vi "Measurement UI.vi"() -> ()   [LabVIEW 2021, in "audio_acMeasurement.lvlib"]
uses:
  audio_acMeasurement.lvlib
panel:
  in  "MeasGraphs":T1(tab)
  out "FreqDomainGraph":cluster{"x0":dbl, "dx":dbl, "magnitude":dbl[]}(graph) caption="AC"
  out "TimeDomainGraph":waveform(dbl)(graph) caption="AC"
  in  "JSONFile":string
  out "Channel":string
  out "Spectrum":dbl[](array[numeric])
  out "df":dbl
  out "f0":dbl
  out "Time domain":dbl[](array[numeric])
  out "dt":dbl
  out "THD+N":dbl
  out "THD":dbl
  out "SNR":dbl
  out "Calculated amplitude":dbl
  out "Calculated frequency":dbl
  out "SFDR":dbl
  out "Dynamic range":dbl
  out "Gain error":dbl
  in  "Analog source resource name":string
  out "MeasTable":string[][](table)
  in  "Filename":string(combo)
  out "Sample rate":u32 caption="SAMPLE RATE" format="%#.6pHz"
  in  "Protocol capture channel":string="0L" caption="CHANNEL"
  in  "Protocol capture resource name":string caption="RESOURCE NAME"
  in  "Protocol settings":string="Protocol settings"
  in  "Analog source":string="Analog source "
  in  "Full scale range":dbl=3.16 caption="FULL SCALE RANGE" format="%.3pV"
  in  "Measurement settings":string="Measurement settings"
  in  "MeasSettingsOptions":i32(listbox)=-1
  in  "MeasSettings":bool
  in  "Protocol":u16(ring) caption="PROTOCOL" items=["I2S"]
  in  "DSGResourceName":tag caption="RESOURCE NAME"
  in  "Weighting filter":T2(ring) caption="WEIGHTING FILTER"
  in  "Number of words":u32=19200 caption="NUMBER OF WORDS"
  in  "Clock rate":u32=12288000 caption="CLOCK RATE" format="%#.6pHz"
  in  "Band stop":dbl=20000.0 caption="BAND STOP" format="%#_6pHz"
  in  "Band start":dbl=20.0 caption="BAND START" format="%#_6pHz"
  in  "Amplitude":dbl=-1.0 caption="AMPLITUDE" format="%#_6pdB"
  in  "Frequency":dbl=1000.0 caption="FREQUENCY" format="%#_6pHz"
  in  "Sensitivity":dbl=0.34762 caption="SENSITIVITY" format="%.5fFS/Pa"
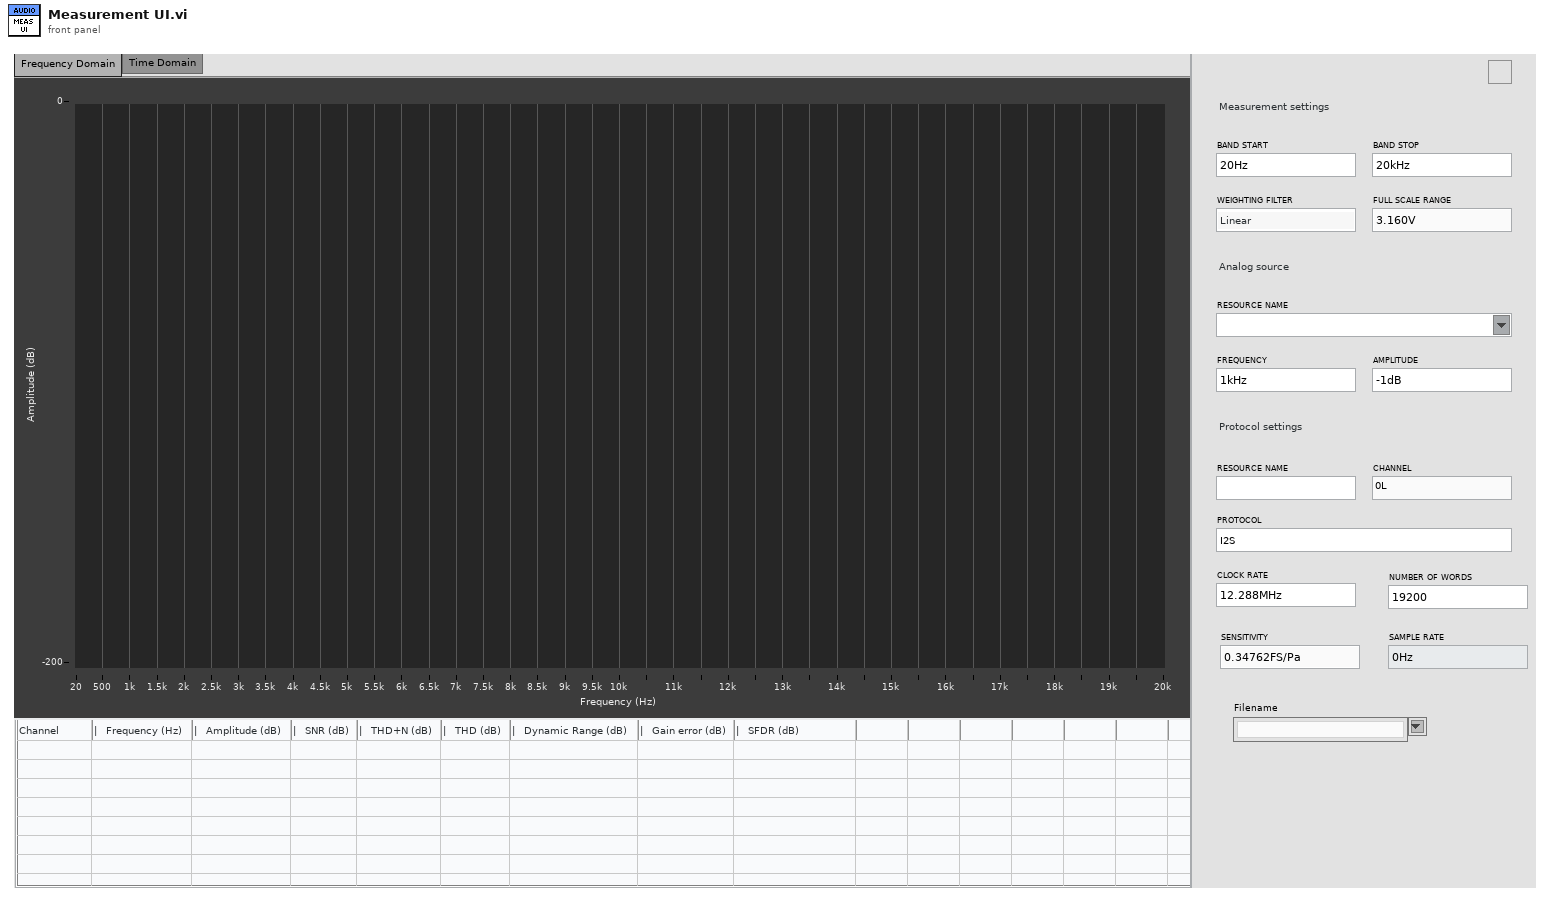
[diagram p1: front panel]
types:
  T1 = enum32{"Frequency Domain", "Time Domain", "Hidden Controls"}
  T2 = enum16{"Linear", "A-Weighting", "B-Weighting", "C-Weighting"}
  T3 = enum16{"open", "replace", "create", "open or create", "replace or create", "replace or create with confirmation"}
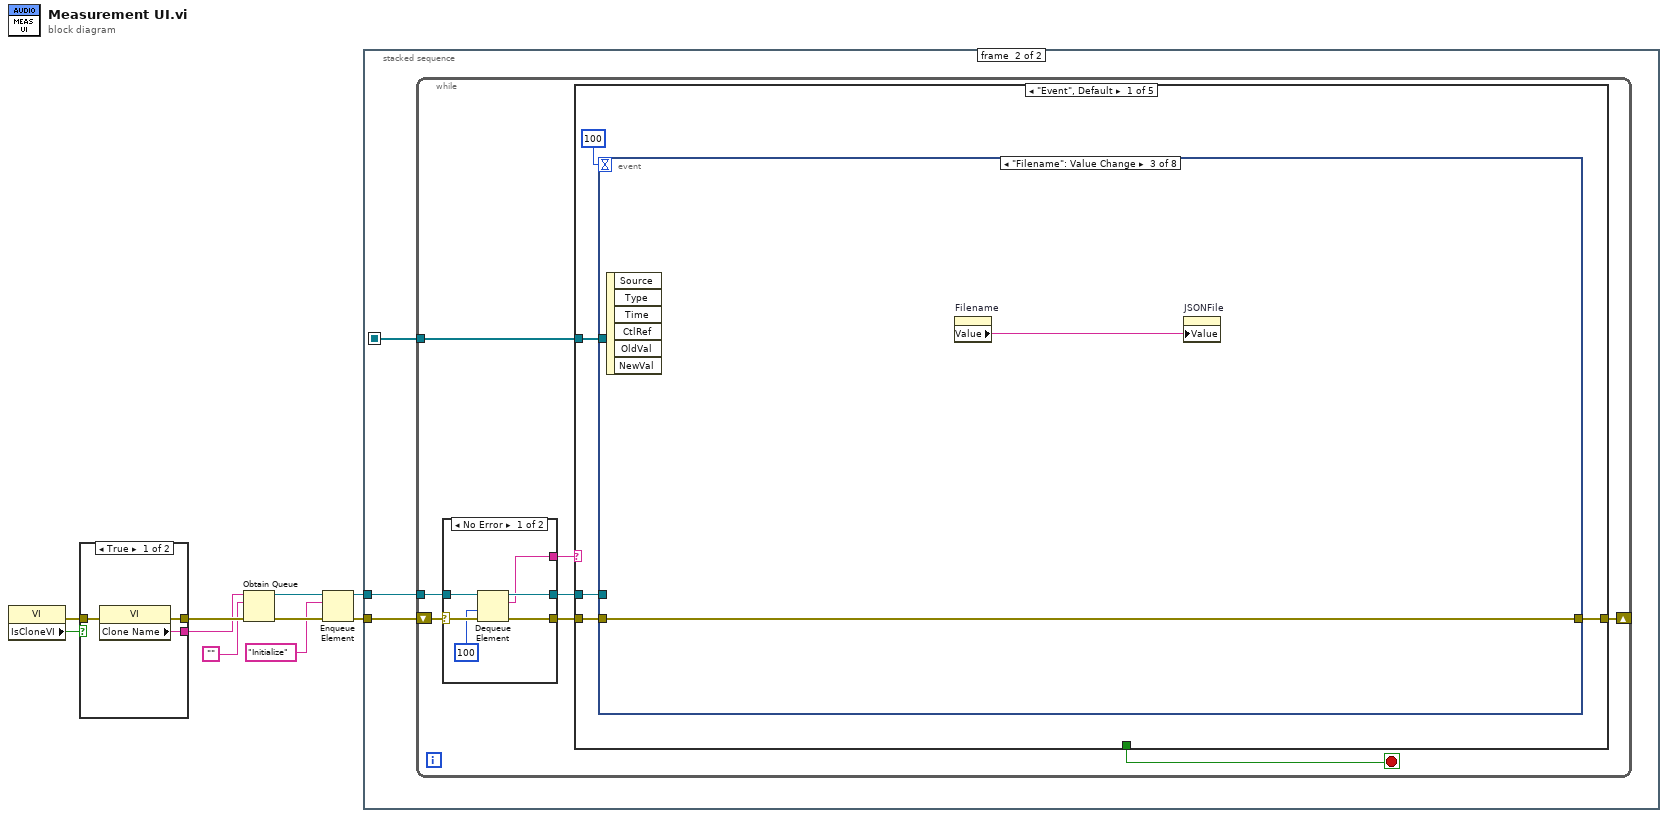
[diagram p0: block diagram]
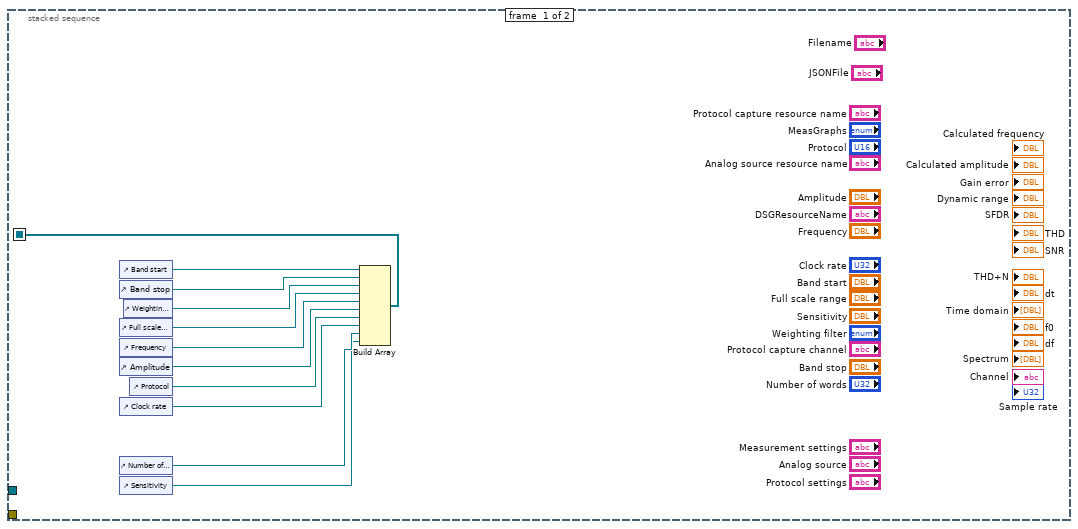
[diagram p2: hidden frame]
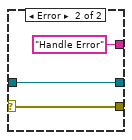
[diagram p3: hidden frame]
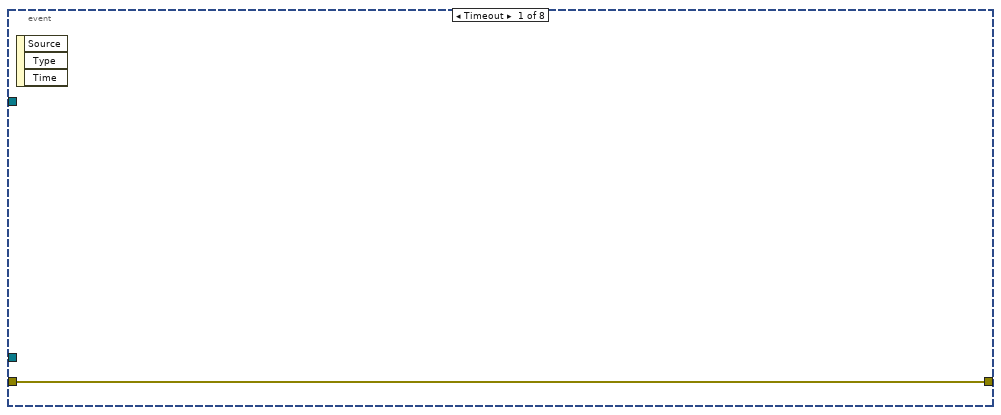
[diagram p4: hidden frame]
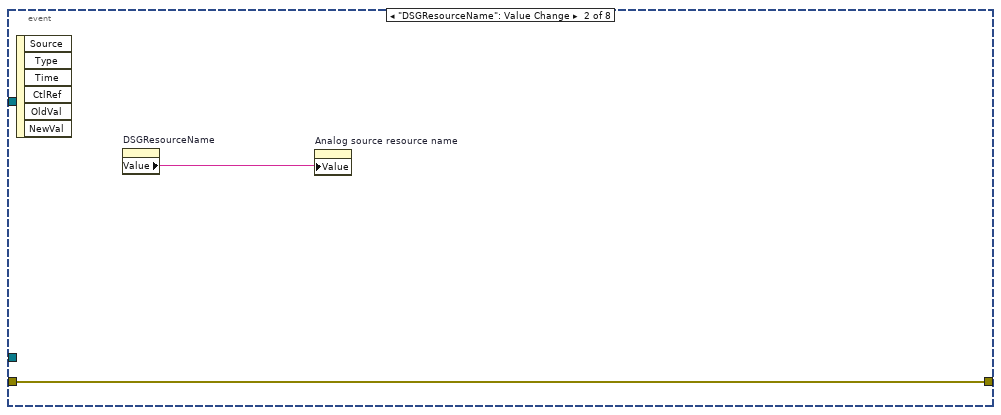
[diagram p5: hidden frame]
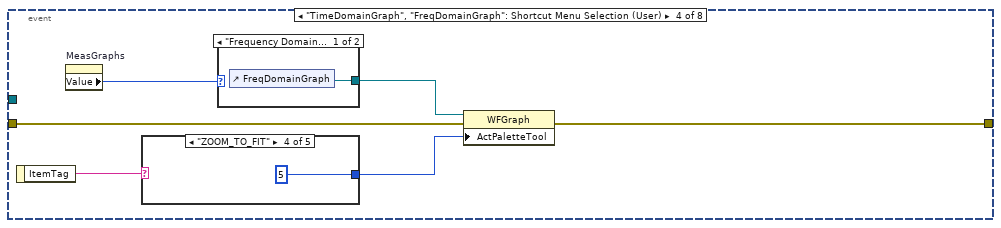
[diagram p6: hidden frame]
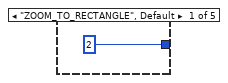
[diagram p7: hidden frame]
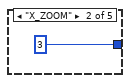
[diagram p8: hidden frame]
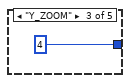
[diagram p9: hidden frame]
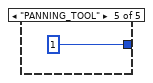
[diagram p10: hidden frame]
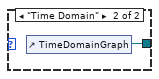
[diagram p11: hidden frame]
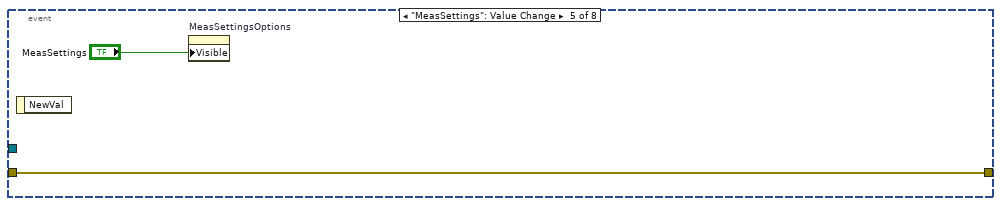
[diagram p12: hidden frame]
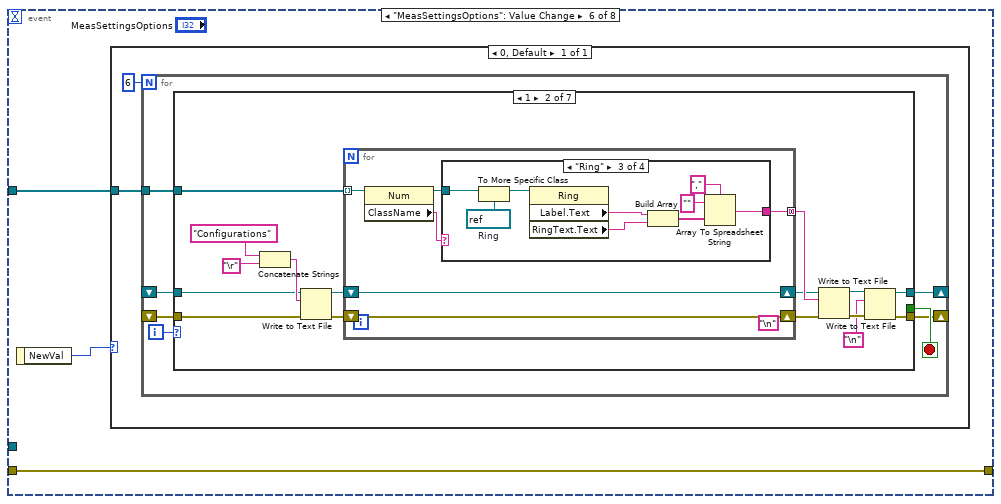
[diagram p13: hidden frame]
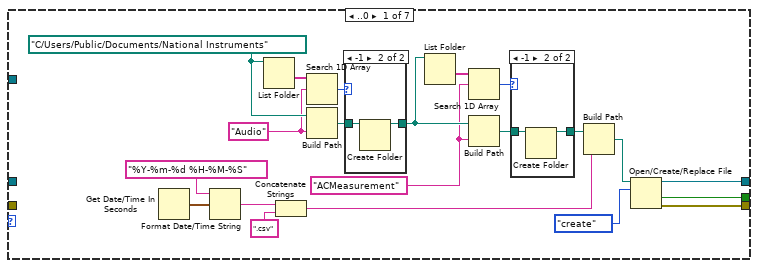
[diagram p14: hidden frame]
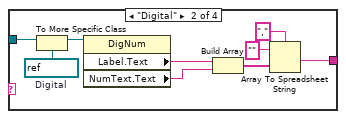
[diagram p18: hidden frame]
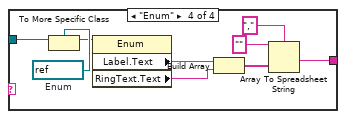
[diagram p19: hidden frame]
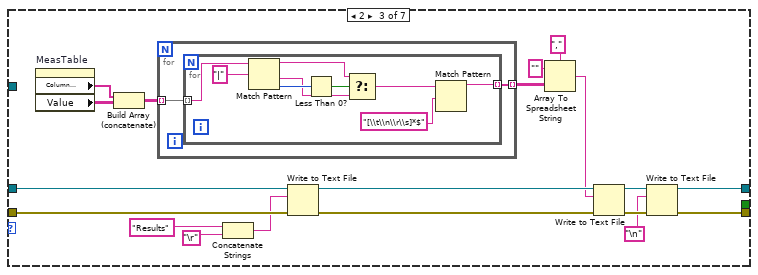
[diagram p20: hidden frame]
diagram:
  n1 = property class="VI"() -> (error out=w1:errorcluster, "IsCloneVI"=w2:bool)  [unwired: 2 in, 1 out]
  n2 = case shown="True" w2 {
    tunnel: [w13 w16] -> w10
    tunnel: [w12 w15] -> w9
    tunnel: w1 -> [w11 w14]
    frame True {
      n3 = property class="VI"(error in=w11) -> (error out=w13:errorcluster, "Clone Name"=w12:string)  [unwired: 1 in, 1 out]
    }
    frame False {
      n4 = property class="VI"(error in=w14) -> (error out=w16:errorcluster, "Name"=w15:string)  [unwired: 1 in, 1 out]
    }
  }
  n5 = Obtain Queue(name (unnamed)=w9, element data type="", error in (no error)=w10) -> (queue out=w6:refnum<queue>, error out=w8:errorcluster)  [unwired: 2 in, 1 out]
  n6 = Enqueue Element(queue=w6, element="Initialize", error in (no error)=w8) -> (queue out=w5:refnum<queue>, error out=w7:errorcluster)  [unwired: 1 in, 1 out]
  n7 = stacked-sequence {
    seq-local: [w24 _] -> [_ w28]
    tunnel: w7 -> [_ w30]
    tunnel: w5 -> [_ w29]
    frame #0 {
      n8 = control-ref of="Band start"() -> (w27:refnum<vi>)
      n9 = control-ref of="Band stop"() -> (w26:refnum<vi>)
      n10 = control-ref of="Full scale range"() -> (w23:refnum<vi>)
      n11 = control-ref of="Frequency"() -> (w20:refnum<vi>)
      n12 = control-ref of="Amplitude"() -> (w19:refnum<vi>)
      n13 = control-ref of="Clock rate"() -> (w22:refnum<vi>)
      n14 = control-ref of="Number of words"() -> (w18:refnum<vi>)
      n15 = control-ref of="Sensitivity"() -> (w17:refnum<vi>)
      n16 = control-ref of="Weighting filter"() -> (w25:refnum<vi>)
      n17 = control-ref of="Protocol"() -> (w21:refnum<vi>)
      n18 = Build Array(w27, w26, w25, w23, w20, w19, w21, w22, w18, w17) -> (w24:refnum<vi>[])
    }
    frame #1 {
      n19 = while {
        shift-right: [w33] -> _
        shift-left: w30 -> [w38]
        tunnel: w29 -> [w36]
        tunnel: w28 -> [w31]
        stop <- w32 stop-if-true
        n20 = case shown="No Error" w38 {
          selector: w38 -> [w44 w47]
          tunnel: [w43 w47] -> w37
          tunnel: w36 -> [w42 w46]
          tunnel: [w41 w46] -> w35
          tunnel: [w40 "Handle Error"] -> w34
          frame No Error {
            n21 = Dequeue Element(queue=w42, timeout in ms (-1)=100, error in (no error)=w44) -> (queue out=w41:refnum<queue>, element=w40:string, error out=w43:errorcluster)  [unwired: 1 out]
          }
          frame Error {
          }
        }
        n22 = case shown="\"Event\", Default" w34 {
          tunnel: w37 -> [w52 w283 w321 w336 w337]
          tunnel: w35 -> [w50 _ _ w334 _]
          tunnel: [w48 w283 w321 w331 w337] -> w33
          tunnel: [_ _ _ TRUE _] -> w32
          tunnel: w31 -> [w49 _ _ _ _]
          frame "Event", Default {
            n23 = event shown="[2] \"Filename\": Value Change" {
              selector: _ -> [_ _ _ _ _ _ _ _]
              dyn-events: _ -> [_ _ _ _ _ _ _ _]
              timeout: 100 -> [_ _ _ _ _ _ _ _]
              tunnel: w52 -> [w53 w54 w56 w59 w71 w75 w267 w273]
              tunnel: w50 -> [_ _ _ _ _ _ _ w271]
              tunnel: [_ _ _ _ w71 _ _ _] -> _
              tunnel: w49 -> [_ _ _ _ _ w73 _ _]
              tunnel: [w53 w54 w56 w60 _ w75 w267 w272] -> w48
              event Timeout {
                n24 = event-data() -> ()  [unwired: 1 in, 3 out]
              }
              event "DSGResourceName": Value Change {
                n25 = event-data() -> ()  [unwired: 1 in, 6 out]
                n26 = property on="DSGResourceName" class="DAQmxName"() -> ("Value"=w55:string)  [unwired: 2 in, 2 out]
                n27 = property on="Analog source resource name" class="Str"("Value"=w55) -> ()  [unwired: 2 in, 2 out]
              }
              event "Filename": Value Change {
                n28 = event-data() -> ()  [unwired: 1 in, 6 out]
                n29 = property on="Filename" class="CmbBox"() -> ("Value"=w57:string)  [unwired: 2 in, 2 out]
                n30 = property on="JSONFile" class="Str"("Value"=w57) -> ()  [unwired: 2 in, 2 out]
              }
              event "TimeDomainGraph", "FreqDomainGraph": Shortcut Menu Selection (User) {
                n31 = event-data() -> ("ItemTag"=w62:string)  [unwired: 1 in]
                n32 = property on="MeasGraphs" class="TabCtl (strict)"() -> ("Value"=w63:T1)  [unwired: 2 in, 2 out]
                n33 = case shown="\"ZOOM_TO_FIT\"" w62 {
                  tunnel: [2 3 4 5 1] -> w58
                  frame "ZOOM_TO_RECTANGLE", Default {
                  }
                  frame "X_ZOOM" {
                  }
                  frame "Y_ZOOM" {
                  }
                  frame "ZOOM_TO_FIT" {
                  }
                  frame "PANNING_TOOL" {
                  }
                }
                n34 = case shown="\"Frequency Domain\", Default" w63 {
                  tunnel: [w69 w70] -> w61
                  frame "Frequency Domain", Default {
                    n35 = control-ref of="FreqDomainGraph"() -> (w69:refnum<vi>)
                  }
                  frame "Time Domain" {
                    n36 = control-ref of="TimeDomainGraph"() -> (w70:refnum<vi>)
                  }
                }
                n37 = property class="WFGraph"(reference=w61, error in=w59, "ActPaletteTool"=w58) -> (error out=w60:errorcluster)  [unwired: 1 out]
              }
              event "MeasSettings": Value Change {
                n38 = event-data() -> ()  [unwired: 1 in, 1 out]
                n39 = property on="MeasSettingsOptions" class="LstBox (strict)"("Visible"="MeasSettings") -> ()  [unwired: 2 in, 2 out]
              }
              event "MeasSettingsOptions": Value Change {
                n40 = event-data() -> ("NewVal"=w74:i32)  [unwired: 1 in]
                n41 = case shown="0, Default" w74 {
                  tunnel: w73 -> [w76]
                  frame 0, Default {
                    n42 = for {
                      N: 6 -> [_]
                      shift-right: [w82] -> _
                      shift-left: _ -> [w81]
                      shift-right: [w80] -> _
                      shift-left: _ -> [w79]
                      tunnel: w76 -> [w78]
                      i -> [w84]
                      stop <- w83 stop-if-true
                      n43 = case shown="1" w84 {
                        tunnel: [w98 _ _ _ _ _ _] -> w83
                        tunnel: [w104 w124 w168 w195 w236 refnum<file> refnum ("refnum out") w266] -> w82
                        tunnel: w81 -> [_ w121 w179 w218 w237 w264 w266]
                        tunnel: [w97 w123 w167 w193 w235 w262 w265] -> w80
                        tunnel: w79 -> [_ w119 w178 w217 w238 w261 w265]
                        tunnel: w78 -> [_ w122 _ _ _ _ _]
                        frame ..0 {
                          w93 = "ACMeasurement" ("prompt")
                          w100 = "Audio" ("prompt")
                          w103 = path "C:/Users/Public/Documents/National Instruments" ("base path")
                          n44 = Get Date/Time In Seconds() -> (seconds since 1Jan1904=w90:timestamp)
                          n45 = Format Date/Time String(time format string (%c)="%Y-%m-%d %H-%M-%S", seconds (now)=w90) -> (date/time string=w89:string)  [unwired: 1 in]
                          n46 = List Folder(path=w103) -> (folder names=w101:string[])  [unwired: 3 in, 3 out]
                          n47 = Concatenate Strings(w89, ".csv" ("string")) -> (w86:string)
                          n48 = Search 1D Array(1D array=w101, element=w100) -> (index of element=w99:i32)  [unwired: 1 in]
                          n49 = Build Path(base path=w103, name or relative path=w100) -> (appended path=w102:path)
                          n50 = case shown="-1" w99 {
                            tunnel: w102 -> [w109 w111]
                            tunnel: [w109 w110] -> w94
                            frame Default {
                            }
                            frame -1 {
                              n51 = Create Folder(path (use dialog)=w111) -> (created path=w110:path)  [unwired: 2 in, 2 out]
                            }
                          }
                          n52 = List Folder(path=w94) -> (folder names=w96:string[])  [unwired: 3 in, 3 out]
                          n53 = Search 1D Array(1D array=w96, element=w93) -> (index of element=w95:i32)  [unwired: 1 in]
                          n54 = Build Path(base path=w94, name or relative path=w93) -> (appended path=w92:path)
                          n55 = case shown="-1" w95 {
                            tunnel: w92 -> [w106 w108]
                            tunnel: [w106 w107] -> w87
                            frame Default {
                            }
                            frame -1 {
                              n56 = Create Folder(path (use dialog)=w108) -> (created path=w107:path)  [unwired: 2 in, 2 out]
                            }
                          }
                          n57 = Build Path(base path=w87, name or relative path=w86) -> (appended path=w85:path)
                          n58 = Open/Create/Replace File(file path (use dialog)=w85, operation (0:open)=T3."create") -> (refnum out=w104:refnum<file>, cancelled=w98:bool, error out=w97:errorcluster)  [unwired: 4 in]
                        }
                        frame 1 {
                          (unwired) "\n"
                          n59 = Concatenate Strings("Configurations" ("format string"), "\r") -> (w125:string)
                          n60 = Write to Text File(file (use dialog)=w121, text=w125, error in=w119) -> (refnum out=w118:refnum<file>, error out=w120:errorcluster)  [unwired: 1 in, 1 out]
                          n61 = for {
                            tunnel: w122 -> [w129] mode=indexing
                            shift-right: [w133] -> w116
                            shift-left: w118 -> [w133]
                            shift-right: [w132] -> w115
                            shift-left: w120 -> [w132]
                            tunnel: [w131] -> w117 mode=concatenating
                            n62 = property class="Num"(reference=w129) -> (reference out=w130:refnum<vi>, "ClassName"=w128:string)  [unwired: 1 in, 1 out]
                            n63 = case shown="\"Ring\"" w128 {
                              tunnel: [_ w137 w147 w156] -> w131
                              tunnel: w130 -> [_ w135 w145 w160]
                              frame Default {
                              }
                              frame "Digital" {
                                w134 = refnum<vi> refnum  # Digital
                                n64 = To More Specific Class(target class=w134, reference=w135) -> (specific class reference=w136:refnum<vi>)  [unwired: 1 in, 1 out]
                                n65 = property class="DigNum"(reference=w136) -> ("Label.Text"=w142:string, "NumText.Text"=w141:string)  [unwired: 1 in, 2 out]
                                n66 = Build Array(w142, w141) -> (w138:string[])
                                n67 = Array To Spreadsheet String(delimiter (Tab)=",", array=w138, 3:"" ("format string")) -> (spreadsheet string=w137:string)
                              }
                              frame "Ring" {
                                w144 = refnum<vi> refnum  # Ring
                                n68 = To More Specific Class(target class=w144, reference=w145) -> (specific class reference=w146:refnum<vi>)  [unwired: 1 in, 1 out]
                                n69 = property class="Ring"(reference=w146) -> ("Label.Text"=w143:string, "RingText.Text"=w151:string)  [unwired: 1 in, 2 out]
                                n70 = Build Array(w143, w151) -> (w148:string[])
                                n71 = Array To Spreadsheet String(delimiter (Tab)=",", array=w148, 3:"" ("format string")) -> (spreadsheet string=w147:string)
                              }
                              frame "Enum" {
                                w159 = refnum<vi> refnum  # Enum
                                n72 = To More Specific Class(target class=w159, reference=w160) -> (specific class reference=w155:refnum<vi>)  [unwired: 1 in, 1 out]
                                n73 = property class="Enum"(reference=w155) -> ("Label.Text"=w154:string, "RingText.Text"=w153:string)  [unwired: 1 in, 2 out]
                                n74 = Build Array(w154, w153) -> (w152:string[])
                                n75 = Array To Spreadsheet String(delimiter (Tab)=",", array=w152, 3:"" ("format string")) -> (spreadsheet string=w156:string)
                              }
                            }
                          }
                          n76 = Write to Text File(file (use dialog)=w116, text=w117, error in=w115) -> (refnum out=w114:refnum<file>, error out=w113:errorcluster)  [unwired: 1 in, 1 out]
                          n77 = Write to Text File(file (use dialog)=w114, text="\n", error in=w113) -> (refnum out=w124:refnum<file>, error out=w123:errorcluster)  [unwired: 1 in, 1 out]
                        }
                        frame 2 {
                          n78 = property on="MeasTable" class="Tbl (strict)"() -> ("Column Headers[]"=w162:string[], "Value"=w161:string[][])  [unwired: 2 in, 2 out]
                          n79 = Build Array (concatenate)(w162, w161) -> (w176:string[][])
                          n80 = for {
                            tunnel: w176 -> [w181] mode=indexing
                            tunnel: [w180] -> w175 mode=indexing
                            n81 = for {
                              tunnel: w181 -> [w183] mode=indexing
                              tunnel: [w182] -> w180 mode=indexing
                              n82 = Match Pattern(string=w183, regular expression="|") -> (before substring=w187:string, after substring=w186:string, offset past match=w189:i32)  [unwired: 1 in, 1 out]
                              n83 = Less Than 0?(x=w189) -> (x < 0?=w188:bool)
                              n84 = Select(t=w187, s=w188, f=w186) -> (s? t:f=w185:string)
                              n85 = Match Pattern(string=w185, regular expression="[\\t\\n\\r\\s]*$") -> (before substring=w182:string)  [unwired: 1 in, 3 out]
                            }
                          }
                          n86 = Concatenate Strings("Results" ("element"), "\r") -> (w163:string)
                          n87 = Write to Text File(file (use dialog)=w179, text=w163, error in=w178) -> (refnum out=w177:refnum<file>, error out=w171:errorcluster)  [unwired: 1 in, 1 out]
                          n88 = Array To Spreadsheet String(delimiter (Tab)=",", array=w175, 3:"" ("format string")) -> (spreadsheet string=w172:string)
                          n89 = Write to Text File(file (use dialog)=w177, text=w172, error in=w171) -> (refnum out=w170:refnum<file>, error out=w169:errorcluster)  [unwired: 1 in, 1 out]
                          n90 = Write to Text File(file (use dialog)=w170, text="\n", error in=w169) -> (refnum out=w168:refnum<file>, error out=w167:errorcluster)  [unwired: 1 in, 1 out]
                        }
                        frame 3 {
                          n91 = property on="FreqDomainGraph" class="WFGraph (strict)"() -> ("Value"=w198:cluster{"x0":dbl, "dx":dbl, "magnitude":dbl[]})  [unwired: 2 in, 2 out]
                          n92 = Concatenate Strings("Frequency Domain" ("string"), "\r") -> (w215:string)
                          n93 = Build Array("Frequency (Hz)", "Amplitude (dB)") -> (w214:string[])
                          n94 = Write to Text File(file (use dialog)=w218, text=w215, error in=w217) -> (refnum out=w211:refnum<file>, error out=w210:errorcluster)  [unwired: 1 in, 1 out]
                          n95 = Unbundle By Name(w198) -> ("dx"=w202:dbl, "x0"=w203:dbl, "magnitude"=w201:dbl[])
                          n96 = Array To Spreadsheet String(delimiter (Tab)=",", array=w214, 3:"" ("format string")) -> (spreadsheet string=w209:string)
                          n97 = Write to Text File(file (use dialog)=w211, text=w209, error in=w210) -> (refnum out=w208:refnum<file>, error out=w207:errorcluster)  [unwired: 1 in, 1 out]
                          n98 = for {
                            tunnel: w201 -> [w222] mode=indexing
                            tunnel: w202 -> [w226]
                            tunnel: w203 -> [w224]
                            tunnel: [w219] -> w204 mode=indexing
                            i -> [w227]
                            n99 = Multiply(x=w227, y=w226) -> (x*y=w225:dbl)
                            n100 = Add(x=w225, y=w224) -> (x+y=w223:dbl)
                            n101 = Format Into String(w223) -> (resulting string=w220:string)  [unwired: 3 in, 1 out]
                            n102 = Format Into String(w222) -> (resulting string=w221:string)  [unwired: 3 in, 1 out]
                            n103 = Build Array(w220, w221) -> (w219:string[])
                          }
                          n104 = Array To Spreadsheet String(delimiter (Tab)=",", array=w204, 3:"" ("format string")) -> (spreadsheet string=w200:string)
                          n105 = Write to Text File(file (use dialog)=w208, text=w200, error in=w207) -> (refnum out=w197:refnum<file>, error out=w196:errorcluster)  [unwired: 1 in, 1 out]
                          n106 = Write to Text File(file (use dialog)=w197, text="\n", error in=w196) -> (refnum out=w195:refnum<file>, error out=w193:errorcluster)  [unwired: 1 in, 1 out]
                        }
                        frame 4 {
                          n107 = property on="TimeDomainGraph" class="WFGraph (strict)"() -> ("Value"=w234:waveform(dbl))  [unwired: 2 in, 2 out]
                          n108 = Concatenate Strings("Time Domain" ("string"), "\r") -> (w250:string)
                          n109 = Write to Text File(file (use dialog)=w237, text=w250, error in=w238) -> (refnum out=w247:refnum<file>, error out=w246:errorcluster)  [unwired: 1 in, 1 out]
                          n110 = Build Array("Time (s)", "Amplitude (V)") -> (w249:string[])
                          n111 = Unbundle By Name(w234) -> ("dt"=w232:dbl, "Y"=w233:dbl[])
                          n112 = Array To Spreadsheet String(delimiter (Tab)=",", array=w249, 3:"" ("format string")) -> (spreadsheet string=w245:string)
                          n113 = Write to Text File(file (use dialog)=w247, text=w245, error in=w246) -> (refnum out=w244:refnum<file>, error out=w243:errorcluster)  [unwired: 1 in, 1 out]
                          n114 = for {
                            tunnel: [w256] -> w240 mode=indexing
                            tunnel: w233 -> [w255] mode=indexing
                            tunnel: w232 -> [w253]
                            i -> [w254]
                            n115 = Multiply(x=w253, y=w254) -> (x*y=w252:dbl)
                            n116 = Format Into String(w252) -> (resulting string=w257:string)  [unwired: 3 in, 1 out]
                            n117 = Format Into String(w255) -> (resulting string=w258:string)  [unwired: 3 in, 1 out]
                            n118 = Build Array(w257, w258) -> (w256:string[])
                          }
                          n119 = Array To Spreadsheet String(delimiter (Tab)=",", array=w240, 3:"" ("format string")) -> (spreadsheet string=w239:string)
                          n120 = Write to Text File(file (use dialog)=w244, text=w239, error in=w243) -> (refnum out=w236:refnum<file>, error out=w235:errorcluster)  [unwired: 1 in, 1 out]
                        }
                        frame 5 {
                          w259 = FALSE ("Visible")
                          n121 = Close File(refnum=w264, error in=w261) -> (error out=w262:errorcluster)  [unwired: 1 out]
                          n122 = property on="MeasSettingsOptions" class="LstBox (strict)"("Visible"=w259, "Value"=-1 ("MeasSettingsOptions")) -> ()  [unwired: 2 in, 2 out]
                          n123 = property on="MeasSettings" class="Bool (strict)"("Value"=w259) -> ()  [unwired: 2 in, 2 out]
                        }
                        frame Default {
                        }
                      }
                    }
                  }
                }
              }
              event Mouse Down {
                w268 = FALSE ("Visible")
                n124 = event-data() -> ()  [unwired: 1 in, 1 out]
                n125 = property on="MeasSettingsOptions" class="LstBox (strict)"("Visible"=w268, "Value"=-1 ("MeasSettingsOptions")) -> ()  [unwired: 2 in, 2 out]
                n126 = property on="MeasSettings" class="Bool (strict)"("Value"=w268) -> ()  [unwired: 2 in, 2 out]
              }
              event Panel Close? {
                n127 = event-data() -> ()  [unwired: 1 in, 4 out]
                n128 = Enqueue Element(queue=w271, element="Exit", error in (no error)=w273) -> (error out=w272:errorcluster)  [unwired: 1 in, 2 out]
                n129 = event-data("Discard?"=TRUE) -> ()  [unwired: 1 in, 1 out]
              }
            }
          }
          frame "Initialize" {
            w281 = string[] ["Export data"] ("Item Names")
            w277 = "<Select Device>"
            n130 = for {
              N: 2 -> [_]
              i -> [w286]
              n131 = case shown="0, Default" w286 {
                tunnel: [w289 w290] -> w287
                frame 0, Default {
                  n132 = control-ref of="FreqDomainGraph"() -> (w289:refnum<vi>)
                }
                frame 1 {
                  n133 = control-ref of="TimeDomainGraph"() -> (w290:refnum<vi>)
                }
              }
              n134 = property class="WFGraph"(reference=w287, "ActPaletteTool"=2 ("Palette:Active Tool")) -> ()  [unwired: 1 in, 2 out]
            }
            n135 = property on="DSGResourceName" class="DAQmxName"("Value"=w277) -> ()  [unwired: 2 in, 2 out]
            n136 = property on="Protocol capture resource name" class="Str"("Value"=w277) -> ()  [unwired: 2 in, 2 out]
            n137 = List Folder(path=path "C:/Users/Public/Documents/National Instruments/Audio/Protocols") -> (filenames=w275:string[])  [unwired: 3 in, 3 out]
            n138 = property on="MeasSettingsOptions" class="LstBox (strict)"("Item Names"=w281, "Value"=-1 ("MeasSettingsOptions"), "Visible"=FALSE, "Disabled Items"=i32[] []) -> ()  [unwired: 2 in, 2 out]
            n139 = for {
              tunnel: w281 -> [_] mode=indexing
              i -> [w285]
              n140 = property on="MeasSettingsOptions" class="LstBox (strict)"("Active Row"=w285, "Cell Height"=30 ("Active Row:Cell Height")) -> ()  [unwired: 2 in, 2 out]
            }
            n141 = property on="Filename" class="CmbBox"("Strings[]"=w275) -> ()  [unwired: 2 in, 2 out]
          }
          frame "Post UI Update" {
            w303 = "|   " ("initial string")
            # "This case will be triggered, after framework updates the User interface with result values."
            n142 = local read "Time domain"() -> (w320:dbl[])
            n143 = local read "Spectrum"() -> (w294:dbl[])
            n144 = local read "df"() -> (w296:dbl)
            n145 = local read "dt"() -> (w319:dbl)
            n146 = local read "f0"() -> (w293:dbl)
            n147 = local read "Calculated frequency"() -> (w306:dbl)
            n148 = local read "Calculated amplitude"() -> (w305:dbl)
            n149 = local read "Dynamic range"() -> (w315:dbl)
            n150 = Bundle By Name("Y"=w320, "dt"=w319) -> (→"TimeDomainGraph":waveform(dbl))  [unwired: 1 in]
            n151 = Bundle(cluster=cluster{"x0":dbl, "dx":dbl, "magnitude":dbl[]} {"x0"=0.0, "dx"=0.0, "magnitude"=[]} ("FreqDomainGraph"), "x0"=w293, "dx"=w296, "magnitude"=w294) -> (→"FreqDomainGraph":cluster{"x0":dbl, "dx":dbl, "magnitude":dbl[]})
            n152 = local read "THD+N"() -> (w316:dbl)
            n153 = local read "Gain error"() -> (w302:dbl)
            n154 = local read "THD"() -> (w317:dbl)
            n155 = local read "SNR"() -> (w304:dbl)
            n156 = local read "SFDR"() -> (w301:dbl)
            n157 = Build Array(w306, w305) -> (w312:dbl[])
            n158 = Build Array(w304, w316, w317, w315) -> (w311:dbl[])
            n159 = for {
              tunnel: w312 -> [w326] mode=indexing
              tunnel: w303 -> [w327]
              tunnel: "%.3f" ("initial string") -> [w328]
              tunnel: [w329] -> w310 mode=indexing
              n160 = Format Into String(format string=w328, initial string=w327, w326) -> (resulting string=w329:string)  [unwired: 1 in, 1 out]
            }
            n161 = for {
              tunnel: w311 -> [w322] mode=indexing
              tunnel: w303 -> [w323]
              tunnel: "%5.1f" ("initial string") -> [w324]
              tunnel: [w325] -> w309 mode=indexing
              n162 = Format Into String(format string=w324, initial string=w323, w322) -> (resulting string=w325:string)  [unwired: 1 in, 1 out]
            }
            n163 = Format Into String(format string="%5.1f" ("initial string"), initial string=w303, w301) -> (resulting string=w299:string)  [unwired: 1 in, 1 out]
            n164 = Format Into String(format string="%5.3f" ("initial string"), initial string=w303, w302) -> (resulting string=w300:string)  [unwired: 1 in, 1 out]
            n165 = local read "Channel"() -> (w291:string)
            n166 = Build Array (concatenate)(w291, w310, w309, w300, w299) -> (w308:string[])
            n167 = Build Array(w308) -> (→"MeasTable":string[][])
          }
          frame "Exit" {
            # "This case is triggered to close the User Interface from framework"
            n168 = Flush Queue(queue=w334, error in (no error)=w336) -> (queue out=w333:refnum<queue>, error out=w332:errorcluster)  [unwired: 1 out]
            n169 = Release Queue(queue=w333, force destroy? (F)=TRUE, error in (no error)=w332) -> (error out=w331:errorcluster)  [unwired: 2 out]
          }
          frame "Handle Error" {
          }
        }
      }
    }
  }
